vi "File.Create Name from SN and Time.vi"(10 "StartTime":timestamp, 11 "SN":string) -> (3 "SN_Time":string)   [LabVIEW 2024]
uses:
  File Utils.lvlib
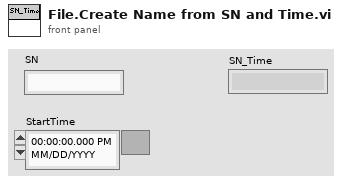
[diagram p1: front panel]
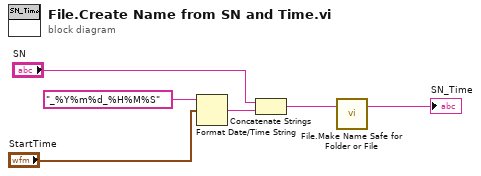
[diagram p0: block diagram]
diagram:
  n1 = Format Date/Time String(time format string (%c)="_%Y%m%d_%H%M%S", seconds (now)="StartTime") -> (date/time string=w6:string)  [unwired: 1 in]
  n2 = Concatenate Strings("SN", w6) -> (w2:string)
  n3 = call "File.Make Name Safe for Folder or File.vi"("File Name"=w2) -> ("Fixed Name"=→"SN_Time":string)  [unwired: 2 in]
